vi "Update UI Interlock.vi"(8 "error in (no error)":errorcluster, 11 "Device Under Test In":refnum<class "Device Under Test.lvclass">) -> (0 "error out":errorcluster, 3 "Device Under Test Out":refnum<class "Device Under Test.lvclass">)   [LabVIEW 2020, in "Device Under Test.lvclass"]
uses:
  Device Under Test.lvclass
  C:/Program Files (x86)/National Instruments/LabVIEW 2020/vi.lib/Astemes/Triarc Framework/Process/Process.lvclass
  <vilib>/Astemes/Triarc Framework/Process/Process.lvclass/Process.ctl
  Device Under Test.lvclass/Device Under Test.ctl
  <vilib>/Utility/error.llb/Clear Errors.vi
  <vilib>/Astemes/Triarc Framework/Process/Private/SubVIs/Handle Debug Data.vi
  <vilib>/Utility/High Resolution Relative Seconds.vi
  <vilib>/Utility/error.llb/Error Cluster From Error Code.vi
  <vilib>/Astemes/Triarc Framework/Process/Process.lvclass
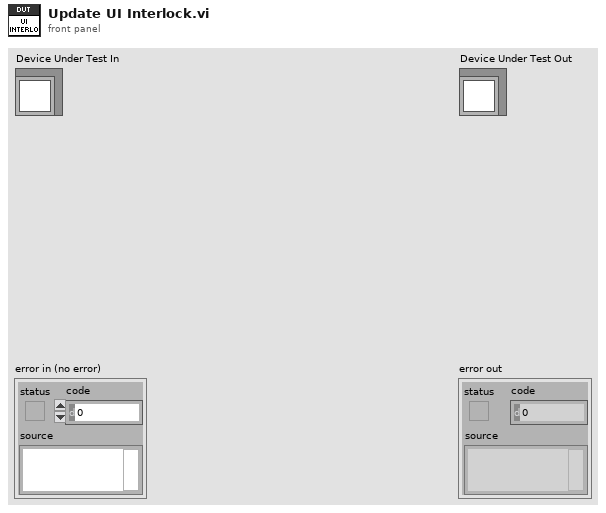
[diagram p1: front panel]
types:
  T1 = enum8{"Enabled", "Disabled", "Disabled and Grayed Out"}
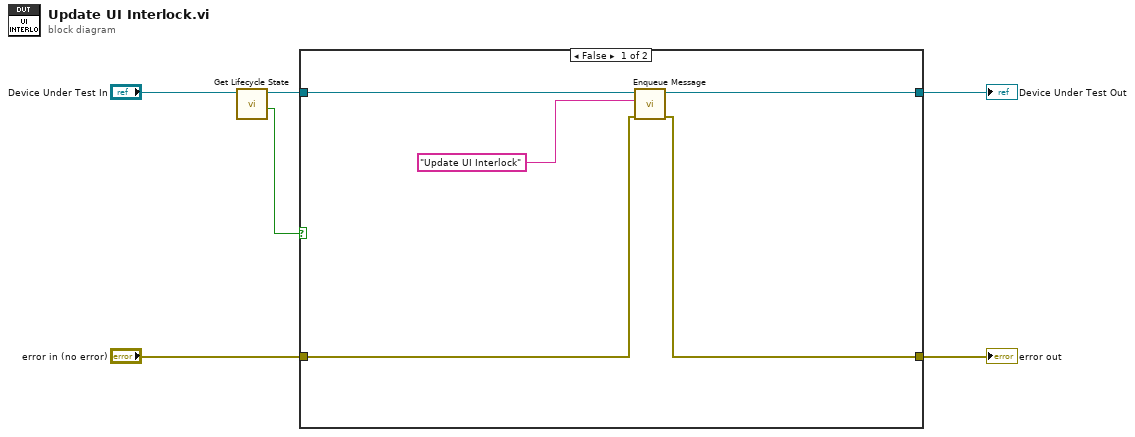
[diagram p0: block diagram]
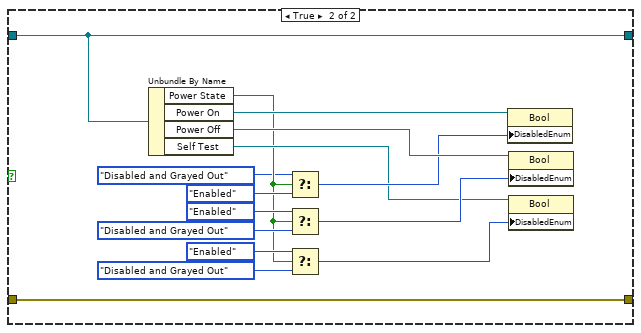
[diagram p2: hidden frame]
diagram:
  n1 = call <vilib>:"Get Lifecycle State.vi"("Process In"="Device Under Test In") -> ("In Process Loop?"=w4:bool, "Process Out"=w5:refnum<class "Device Under Test.lvclass">)  [unwired: 7 in, 2 out]
  n2 = case shown="False" w4 {
    tunnel: w5 -> [w11 w13]
    tunnel: [w10 w13] -> w3
    tunnel: [w8 w12] -> w2
    tunnel: "error in (no error)" -> [w9 w12]
    frame False {
      n3 = call <vilib>:"Enqueue Message.vi"("error in (no error)"=w9, "Message"="Update UI Interlock", "Process In"=w11) -> ("error out"=w8:errorcluster, "Process Out"=w10:refnum<class "Device Under Test.lvclass">)  [unwired: 7 in]
    }
    frame True {
      n4 = Unbundle By Name(w13) -> ("Power State"=w15:bool, "Power On"=w16:refnum<vi>, "Power Off"=w21:refnum<vi>, "Self Test"=w17:refnum<vi>)
      n5 = Select(t=T1."Disabled and Grayed Out" ("Disabled"), s=w15, f=T1."Enabled" ("Disabled")) -> (s? t:f=w20:T1)
      n6 = Select(t=T1."Enabled" ("Disabled"), s=w15, f=T1."Disabled and Grayed Out" ("Disabled")) -> (s? t:f=w19:T1)
      n7 = Select(t=T1."Enabled" ("Disabled"), s=w15, f=T1."Disabled and Grayed Out" ("Disabled")) -> (s? t:f=w18:T1)
      n8 = property class="Bool"(reference=w16, "DisabledEnum"=w20) -> ()  [unwired: 1 in, 2 out]
      n9 = property class="Bool"(reference=w21, "DisabledEnum"=w19) -> ()  [unwired: 1 in, 2 out]
      n10 = property class="Bool"(reference=w17, "DisabledEnum"=w18) -> ()  [unwired: 1 in, 2 out]
    }
  }
  "error out" <- w2
  "Device Under Test Out" <- w3
